vi "Test Native Input Criterion Control.vi"() -> ()   [LabVIEW 2020]
uses:
  Controls/Input Criterion/Input Criterion.xctl
  Controls/Input Criteria Table/Input Criteria Table.xctl
  Digital Input VIs/Tosca-Input Criterion.ctl
  epl-vi-lib/Utility VIs/Type Defs/Logic State.ctl
panel:
  out "NewVal":T3
  in  "stop":bool
  in  "Input Criteria Table":T3(xcontrol)
  in  "Input Criterion":T4(xcontrol)
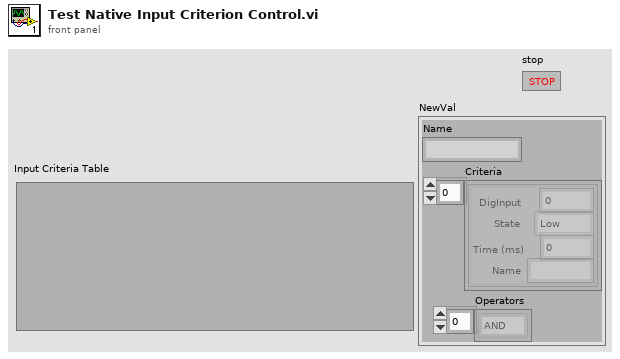
[diagram p1: front panel]
types:
  T1 = typedef "Tosca-Input Criterion.ctl" = cluster{"DigInput":i32, "State":T2, "Time (ms)":i32, "Name":string}
  T2 = typedef "Logic State.ctl" = enum16{"Low", "High", "Rising", "Falling"}
  T3 = cluster{"Name":string, "Criteria":T1[], "Operators":enum16{"AND", "OR"}[]}
  T4 = cluster{"Criterion":T1, "Operator":i16, "visible":bool}
  T5 = typedef "Input Criterion.xctl/Events.ctl" = cluster{"Generic":refnum<user-event>, "Operator":refnum<user-event>, "Criterion":refnum<user-event>}
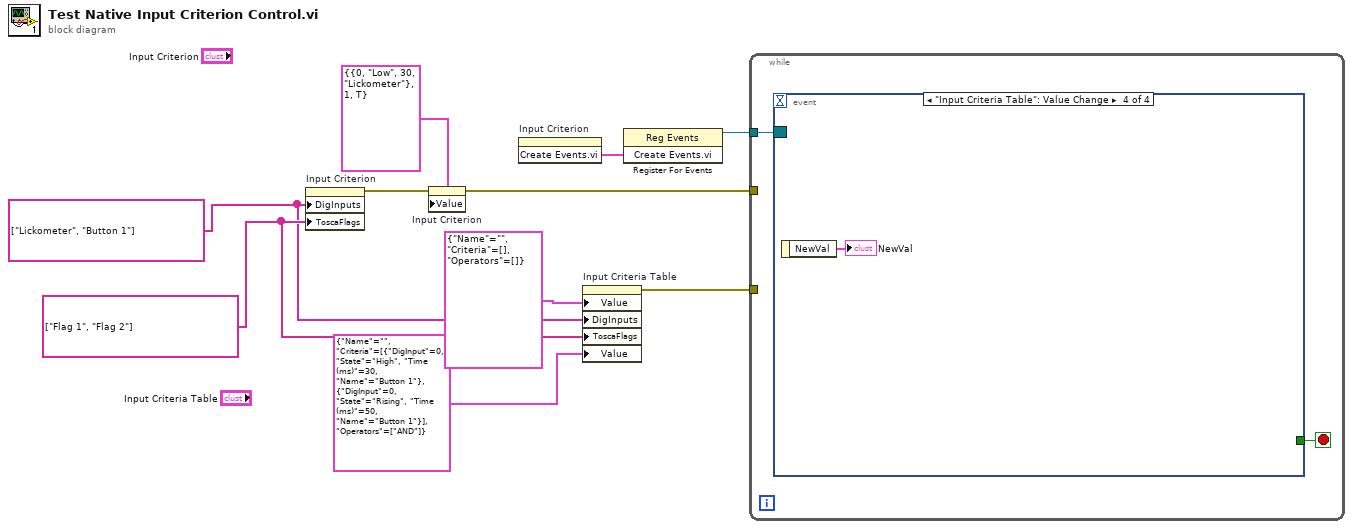
[diagram p0: block diagram]
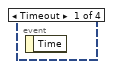
[diagram p2: hidden frame]
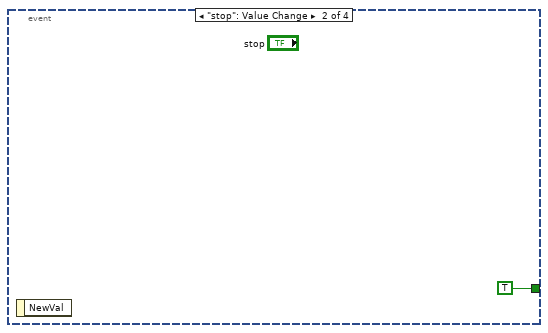
[diagram p3: hidden frame]
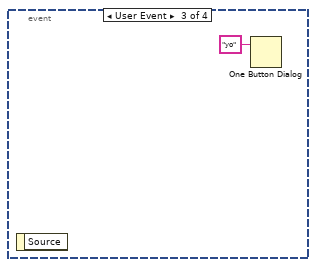
[diagram p4: hidden frame]
diagram:
  w10 = string[] ["Flag 1", "Flag 2"]
  w6 = string[] ["Lickometer", "Button 1"]
  n1 = property on="Input Criterion" class="Criterion (strict)"("DigInputs"=w6, "ToscaFlags"=w10) -> (error out=w8:errorcluster)  [unwired: 2 in, 1 out]
  n2 = property on="Input Criterion" class="Criterion (strict)"(error in=w8, "Value"=cluster{"Criterion":T1, "Operator":i16, bool} {"Criterion"={"DigInput"=0, "State"=enum."Low", "Time (ms)"=30, "Name"="Lickometer"}, "Operator"=1, TRUE} ("Input Criterion")) -> (error out=w4:errorcluster)  [unwired: 1 in, 1 out]
  n3 = invoke on="Input Criterion" class="Criterion (strict)" method="Create Events.vi"() -> ("Create Events.vi"=w2:T5)  [unwired: 3 in, 2 out]
  n4 = property on="Input Criteria Table" class="Input Criteria Table (strict)"("Value"=T3 {"Name"="", "Criteria"=[], "Operators"=[]} ("Input Criteria Table"), "DigInputs"=w6, "ToscaFlags"=w10, "Value"=T3 {"Name"="", "Criteria"=[{"DigInput"=0, "State"=enum."High", "Time (ms)"=30, "Name"="Button 1"}, {"DigInput"=0, "State"=enum."Rising", "Time (ms)"=50, "Name"="Button 1"}], "Operators"=[enum."AND"]} ("Input Criteria Table")) -> (error out=w3:errorcluster)  [unwired: 2 in, 1 out]
  n5 = register-events(w2) -> (reference out=w1:refnum<event-registration>)  [unwired: 2 in, 1 out]
  n6 = while {
    tunnel: w4 -> [_]
    tunnel: w3 -> [_]
    tunnel: w1 -> [w11]
    stop <- w12 stop-if-true
    n7 = event shown="[3] \"Input Criteria Table\": Value Change" {
      selector: w11 -> [_ _ _ _]
      dyn-events: _ -> [_ _ _ _]
      timeout: _ -> [_ _ _ _]
      tunnel: [_ TRUE _ _] -> w12
      event Timeout {
        n8 = event-data() -> ()  [unwired: 1 in, 1 out]
      }
      event "stop": Value Change {
        n9 = event-data() -> ()  [unwired: 1 in, 1 out]
      }
      event User Event {
        n10 = event-data() -> ()  [unwired: 1 in, 1 out]
        n11 = One Button Dialog(message="yo") -> ()  [unwired: 1 in, 1 out]
      }
      event "Input Criteria Table": Value Change {
        n12 = event-data() -> ("NewVal"=→"NewVal":T3)  [unwired: 1 in]
      }
    }
  }
